vi "Initialize.vi"(8 "error in (no error)":errorcluster, 10 "Array of Hardware":refnum<class "Hardware.lvclass">[](array[class]), 11 "CCD monitor in":refnum<class "CCD monitor.lvclass">) -> (0 "error out":errorcluster, 3 "CCD monitor out":refnum<class "CCD monitor.lvclass">)   [LabVIEW 2016, in "CCD monitor.lvlib" / "CCD monitor.lvclass"]
uses:
  <userlib>/Common Components/Hardware/Abstract System/Monitor/CCD monitor.lvclass
  <userlib>/Common Components/Hardware/Abstract Hardware/Hardware.lvclass
  <userlib>/Common Components/Hardware/CCD/CCD/CCD.lvclass
  <userlib>/Common Components/Hardware/Abstract System/Monitor/CCD monitor.lvclass/CCD monitor.ctl
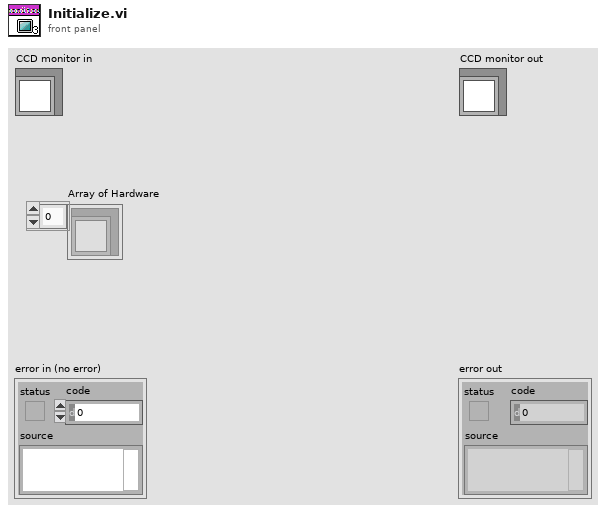
[diagram p1: front panel]
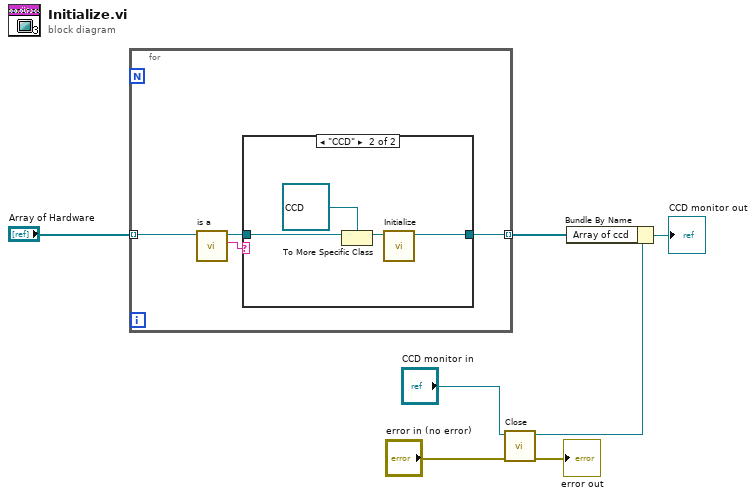
[diagram p0: block diagram]
diagram:
  n1 = for {
    tunnel: "Array of Hardware" -> [w11] mode=indexing
    tunnel: [w8] -> w4 mode=indexing
    n2 = call-dynamic "is a.vi"("Hardware in"=w11) -> ("is a"=w10:string, "Hardware out"=w9:refnum<class "Hardware.lvclass">)  [unwired: 8 in, 1 out]
    n3 = case shown="\"CCD\"" w10 {
      tunnel: w9 -> [_ w15]
      tunnel: [_ w12] -> w8
      frame Default {
      }
      frame "CCD" {
        n4 = To More Specific Class(target class=refnum<class "CCD.lvclass"> refnum ("Hardware.lvlib:CCD.lvlib:CCD.lvclass"), reference=w15) -> (specific class reference=w13:refnum<class "CCD.lvclass">)  [unwired: 1 in, 1 out]
        n5 = call-dynamic "Initialize.vi"("CCD in"=w13) -> ("CCD out"=w12:refnum<class "CCD.lvclass">)  [unwired: 9 in, 1 out]
      }
    }
  }
  n6 = call <userlib>:"Close.vi"("error in (no error)"="error in (no error)", "CCD monitor in"="CCD monitor in") -> ("error out"=→"error out":errorcluster, "CCD monitor out"=w5:refnum<class "CCD monitor.lvclass">)  [unwired: 8 in]
  n7 = Bundle By Name(cluster=w5, "Array of ccd"=w4) -> (→"CCD monitor out":refnum<class "CCD monitor.lvclass">)
